vi "Set Boolean Trigger.vi"(7 "Trigger Direction":T1, 8 "error in (no error)":errorcluster, 10 "Boolean Trigger":T2, 11 "Item Ref in":T3 format="%.0x") -> (0 "error out":errorcluster, 3 "Item Ref out":T3 format="%.0x")   [LabVIEW 2012, in "Waveform Data Logger Shared.lvlib"]
uses:
  Waveform Data Logger Shared.lvlib
  <vilib>/NI Veristand/Custom Device API/Custom Device Item Ref.ctl
  Types/Boolean Trigger.ctl
  Types/Trigger Direction.ctl
  Globals/Property Strings.vi
  <vilib>/NI Veristand/Custom Device API/Set Item Property (Double).vi
  <vilib>/NI Veristand/Custom Device API/Set Item Property (U16).vi
  <vilib>/NI VeriStand/Custom Device API/Custom Device API.lvlib
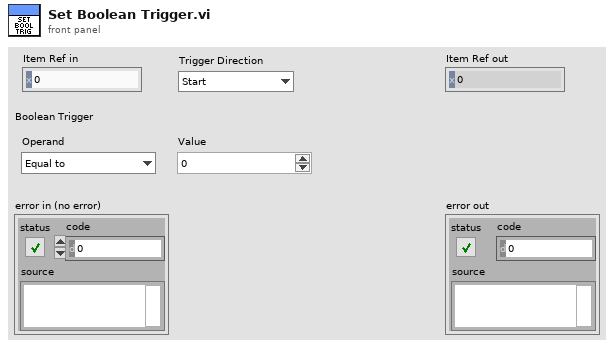
[diagram p1: front panel]
types:
  T1 = typedef "Waveform Data Logger Shared.lvlib/Trigger Direction.ctl" = enum16{"Start", "Stop"}
  T2 = typedef "Waveform Data Logger Shared.lvlib/Boolean Trigger.ctl" = cluster{"Value":dbl, "Operand":enum16{"Equal to", "Not equal to", "Less than", "Less than or equal", "Greater than", "Greater than or equal"}}
  T3 = typedef "Custom Device API.lvlib/Custom Device Item Ref.ctl" = u64
  T4 = enum16{"Equal to", "Not equal to", "Less than", "Less than or equal", "Greater than", "Greater than or equal"}
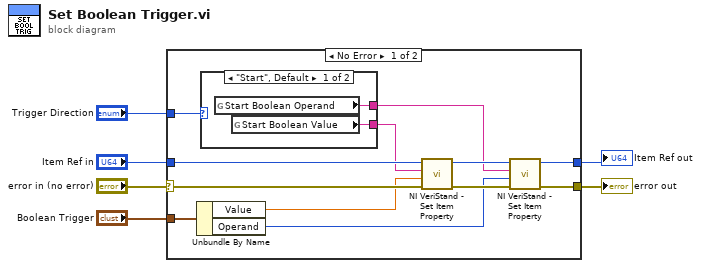
[diagram p0: block diagram]
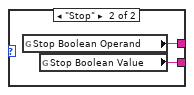
[diagram p2: hidden frame]
diagram:
  n1 = case shown="No Error" "error in (no error)" {
    selector: "error in (no error)" -> [w12 w23]
    tunnel: [w18 w24] -> w6
    tunnel: [w17 w23] -> w5
    tunnel: "Item Ref in" -> [w14 w24]
    tunnel: "Boolean Trigger" -> [w13 _]
    tunnel: "Trigger Direction" -> [w11 _]
    frame No Error {
      n2 = Unbundle By Name(w13) -> ("Value"=w10:dbl, "Operand"=w9:T4)
      n3 = case shown="\"Start\", Default" w11 {
        tunnel: [w20 w22] -> w7
        tunnel: [w19 w21] -> w8
        frame "Start", Default {
          n4 = global read "Property Strings.vi" "Start Boolean Operand"() -> (w20:string)
          n5 = global read "Property Strings.vi" "Start Boolean Value"() -> (w19:string)
        }
        frame "Stop" {
          n6 = global read "Property Strings.vi" "Stop Boolean Operand"() -> (w22:string)
          n7 = global read "Property Strings.vi" "Stop Boolean Value"() -> (w21:string)
        }
      }
      n8 = call-poly <vilib>:"NI VeriStand - Set Item Property.vi"("error in (no error)"=w12, "Value"=w10, "Property Name"=w8, "Item Ref in"=w14) -> ("error out"=w16:errorcluster, "Item Ref out"=w15:T3)  [unwired: 5 in, 1 out]
      n9 = call-poly <vilib>:"NI VeriStand - Set Item Property.vi"("error in (no error)"=w16, "Value"=w9, "Property Name"=w7, "Item Ref in"=w15) -> ("error out"=w17:errorcluster, "Item Ref out"=w18:T3)  [unwired: 5 in, 1 out]
    }
    frame Error {
    }
  }
  "Item Ref out" <- w6
  "error out" <- w5
